vi "While Loop.vi"() -> ()   [LabVIEW 2015]
panel:
  out "Boolean":bool
  out "Thermometer":dbl(slide) scale=0.0..100.0
  in  "Numeric":i32=4
  out "Tank":u32(slide) scale=0.0..10.0
  out "Iterasi":u32
  in  "Reset":bool
  out "Output":dbl
  out "Current Data":dbl
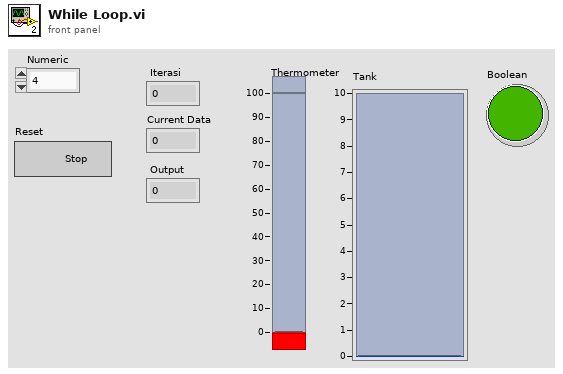
[diagram p1: front panel]
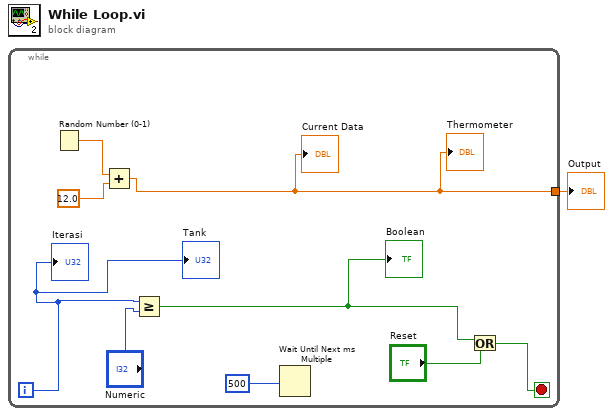
[diagram p0: block diagram]
diagram:
  n1 = while {
    tunnel: [w3] -> w1
    i -> [w4]
    stop <- w7 stop-if-true
    n2 = Random Number (0-1)() -> (number: 0 to 1=w9:dbl)
    n3 = Add(x=w9, y=12.0) -> (x+y=w3:dbl)
    "Current Data" <- w3
    "Thermometer" <- w3
    n4 = Greater Or Equal?(x=w4, y="Numeric") -> (x >= y?=w2:bool)
    "Boolean" <- w2
    n5 = Wait Until Next ms Multiple(millisecond multiple=500) -> ()  [unwired: 1 out]
    n6 = Or(x=w2, y="Reset") -> (x .or. y?=w7:bool)
    "Iterasi" <- w4
    "Tank" <- w4
  }
  "Output" <- w1
